vi "Lissajoust Figures.vi"() -> ()   [LabVIEW 2017]
doc: "This VI uses Express VIs to generate Lissajous figures in order to simulate an oscilloscope."
uses:
  <vilib>/express/express arith-compare/Formula/XNode/ExpressFormulaBlockNode.xnode
panel:
  in  "?":bool
  in  "?":i8(slide) scale=0.0..10.0
  in  "Slide":i8(slide) scale=0.0..10.0
  in  "Trim":dbl(slide) scale=-1.0..1.0
  out "?":cluster{"Y":dbl[], "Y":dbl[]}[](graph)
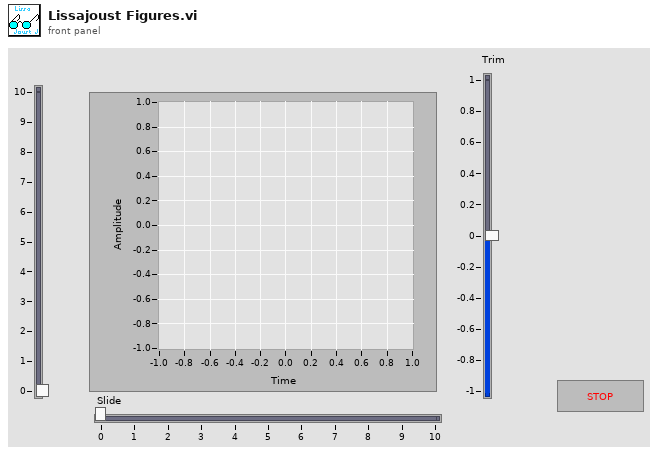
[diagram p1: front panel]
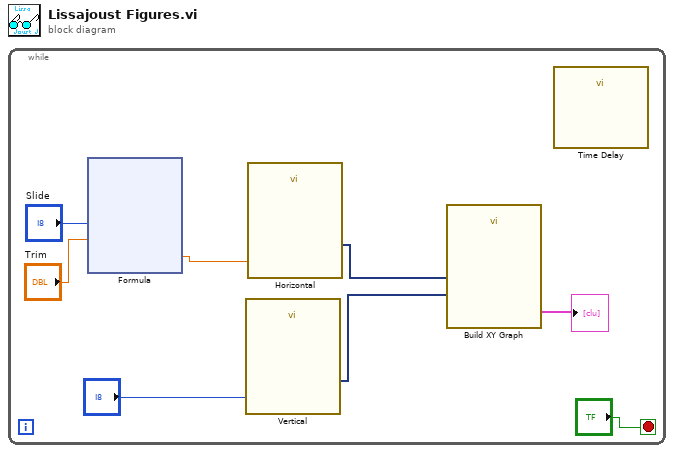
[diagram p0: block diagram]
diagram:
  n1 = while {
    stop <- "?" stop-if-true
    n2 = xnode "Formula"("Slide"="Slide", "Trim"="Trim") -> ("Result"=w6:dbl)  [unwired: 1 in, 1 out]
    n3 = call "Vertical"("Frequency"="?") -> ("Sine"=w3:dynamicdata)  [unwired: 13 in, 1 out]
    n4 = call "Horizontal"("Frequency"=w6) -> ("Sine"=w4:dynamicdata)  [unwired: 13 in, 1 out]
    n5 = call "Build XY Graph"("Y Input"=w3, "X Input"=w4) -> ("XY Graph"=→"?":cluster{"X":dbl[], "Y":dbl[]}[])  [unwired: 8 in, 1 out]
    n6 = call "Time Delay"() -> ()  [unwired: 11 in, 1 out]
  }
